vi "test6-AsteriskWildcardStatusRegistration.vi"(8 "error in (no error)":errorcluster, 11 "TestCase in":refnum<class "testcase-CSMBroadcast.lvclass">) -> (0 "error out":errorcluster, 3 "TestCase out":refnum<class "testcase-CSMBroadcast.lvclass">)   [LabVIEW 2017, in "testcase-CSMBroadcast.lvclass"]
uses:
  testcase-CSMBroadcast.lvclass
  0c20cacf-7d77-4f8e-aec5-f22e7d09936d.vi
  26de337d-8090-412f-9da5-e117a55d4726.vi
  de10340a-d592-45ad-b055-7fa7b377c551.vi
  e3eae2f8-d8ce-4adb-8167-9a417250fce1.vi
  a4d00e00-a9ed-4631-bf53-269bf71f16fc.vi
  src/user.lib/_NEVSTOP/Communicable State Machine(CSM)/AdvanceAPI/CSM - Revert Arguments-Safe String.vi
  src/user.lib/_NEVSTOP/Communicable State Machine(CSM)/_Shared/Trim Single-line Text.vi
  src/user.lib/_NEVSTOP/Communicable State Machine(CSM)/AdvanceAPI/CSM - Make String Arguments Safe.vi
  src/user.lib/_NEVSTOP/Communicable State Machine(CSM)/AdvanceAPI/CSM - Break Down Multiple States String.vi
  src/user.lib/_NEVSTOP/Communicable State Machine(CSM)/AdvanceAPI/CSM - Compact Multiple States.vi
  src/user.lib/_NEVSTOP/Communicable State Machine(CSM)/AdvanceAPI/CSM - Keywords.vi
  src/user.lib/_NEVSTOP/Communicable State Machine(CSM)/AdvanceAPI/CSM - Set Module Attribute.vi
  src/user.lib/_NEVSTOP/Communicable State Machine(CSM)/AdvanceAPI/CSM - Get Module Attribute.vi
  <vilib>/addons/_JKI Toolkits/VI Tester/TestCase.llb/TestCase.lvclass
  src/user.lib/_NEVSTOP/Communicable State Machine(CSM)/Communicable State Machine.lvlib
  C:/Program Files (x86)/National Instruments/LabVIEW 2017/vi.lib/addons/_JKI Toolkits/VI Tester/TestCase.llb/TestCase.lvclass
panel:
  out "Execution Times":i32
  out "State History":string
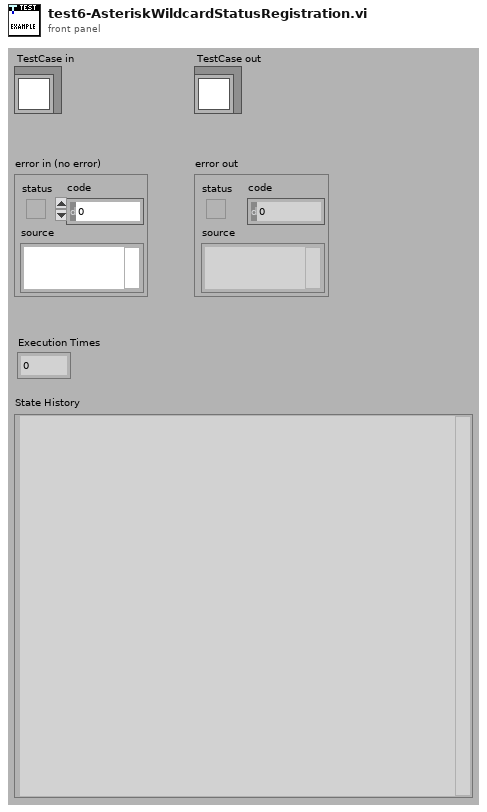
[diagram p1: front panel]
types:
  T1 = enum32{"Invalid", "Standard", "Closed", "Hidden", "Minimized", "Maximized"}
  T2 = enum32{"invalid app kind", "Development System", "Run Time System", "Student Edition", "Embedded LabVIEW", "Evaluation", "Custom"}
  T3 = typedef "Communicable State Machine.lvlib/_CSM_Response Source Message.ctl" = cluster{"‘State":string, "’Arguments":string, "’Error":errorcluster}
  T4 = cluster{"Current VI Reference":refnum<vi>, "Close Panel on Exit?":bool}
  T5 = cluster{"Core":cluster{"Current VI Reference":refnum<vi>, "Close Panel on Exit?":bool}, "Your Boolean data":bool, "Your string data":string, "TestData":i32}
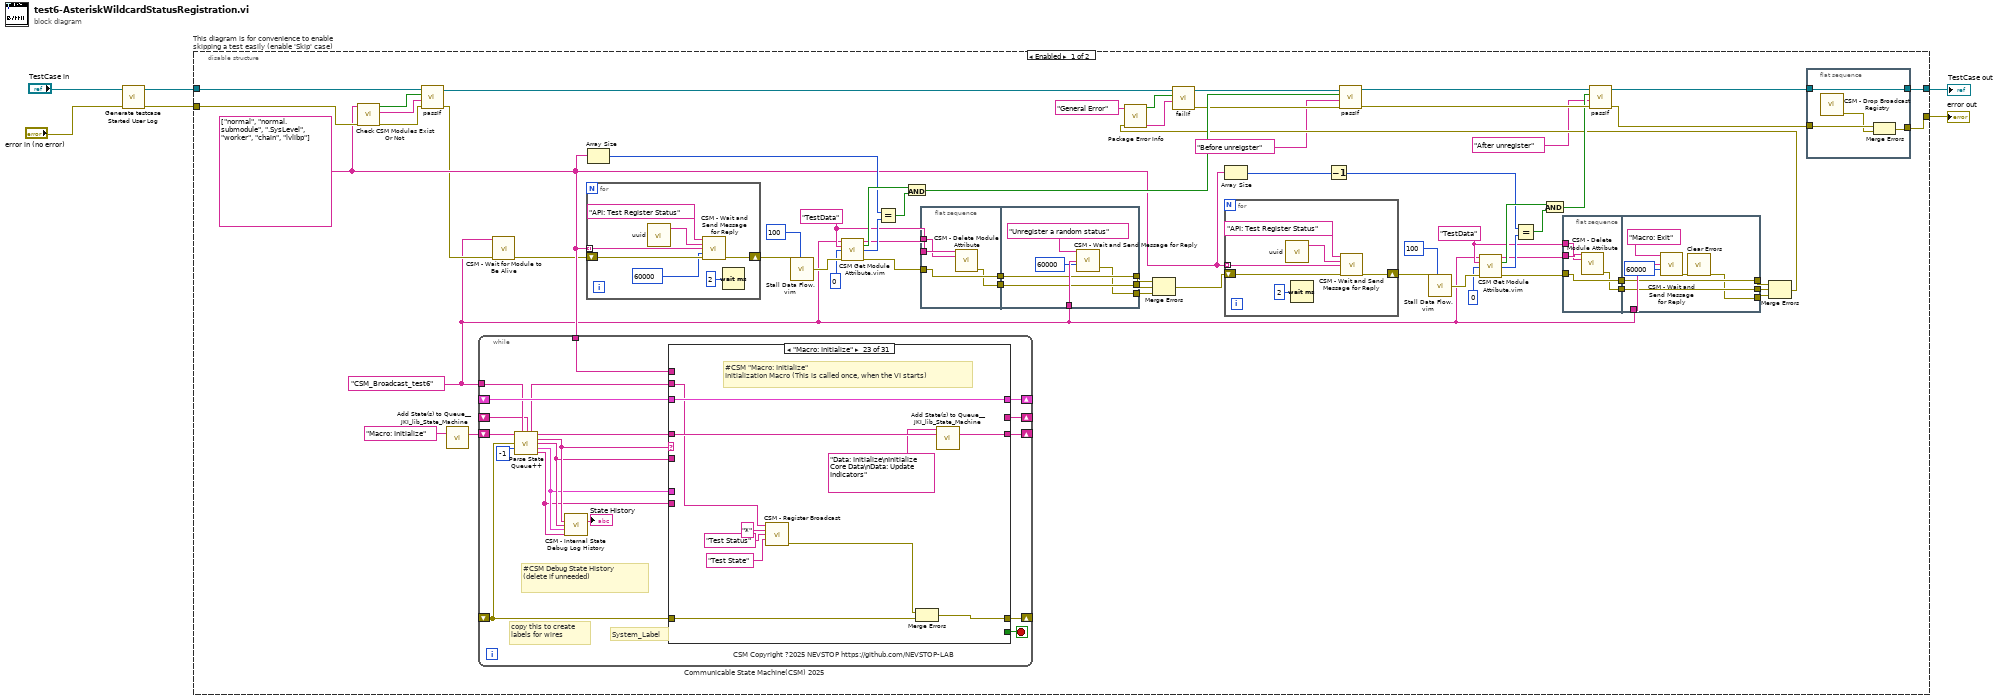
[diagram p0: block diagram]
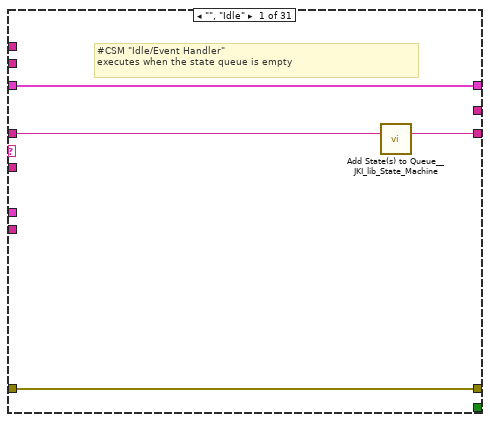
[diagram p2: hidden frame]
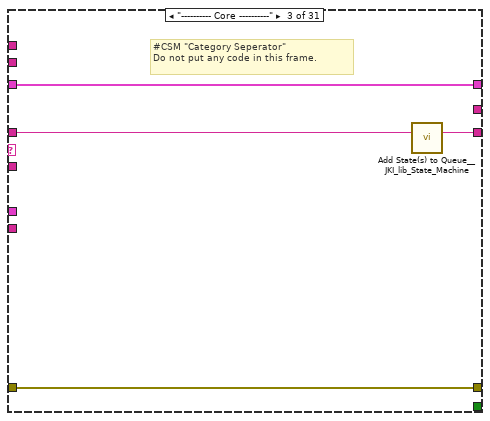
[diagram p4: hidden frame]
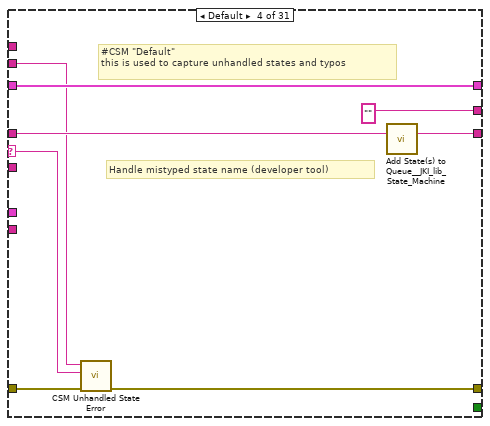
[diagram p5: hidden frame]
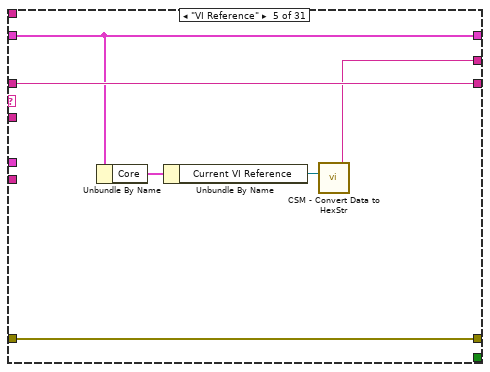
[diagram p6: hidden frame]
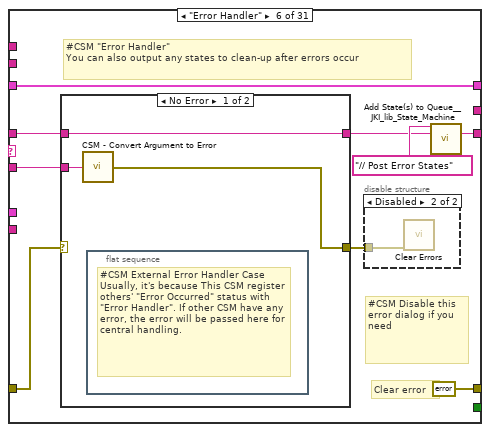
[diagram p7: hidden frame]
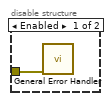
[diagram p8: hidden frame]
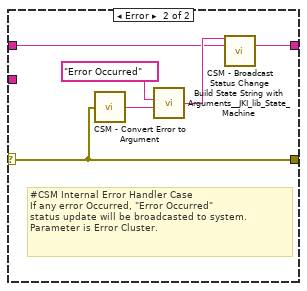
[diagram p9: hidden frame]
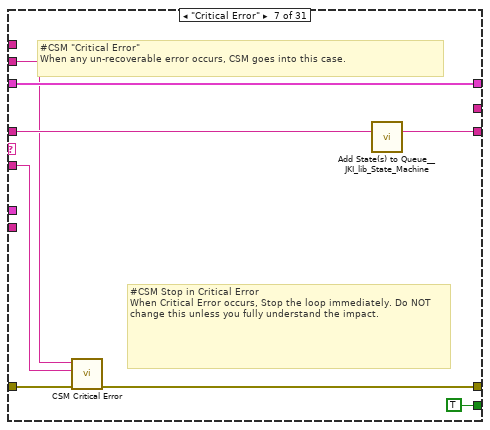
[diagram p10: hidden frame]
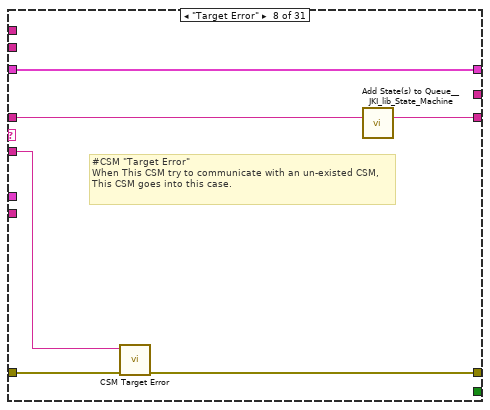
[diagram p11: hidden frame]
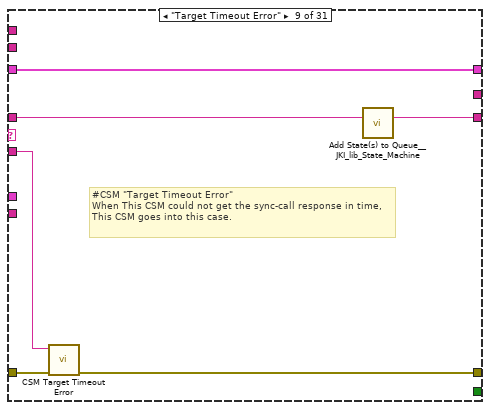
[diagram p12: hidden frame]
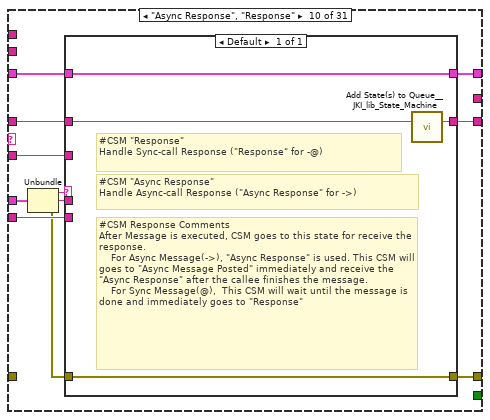
[diagram p13: hidden frame]
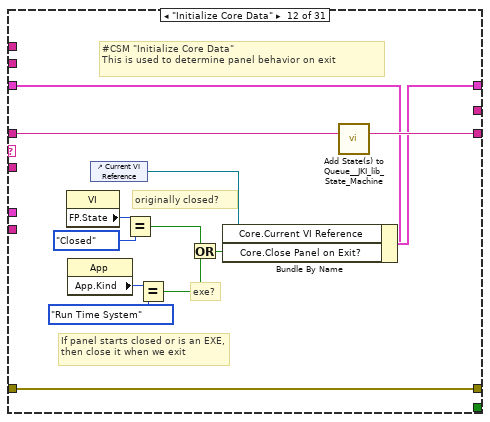
[diagram p15: hidden frame]
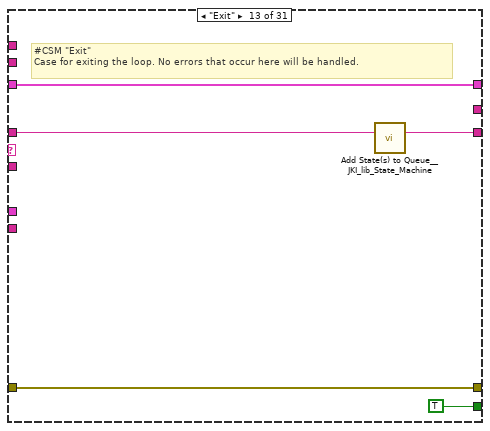
[diagram p16: hidden frame]
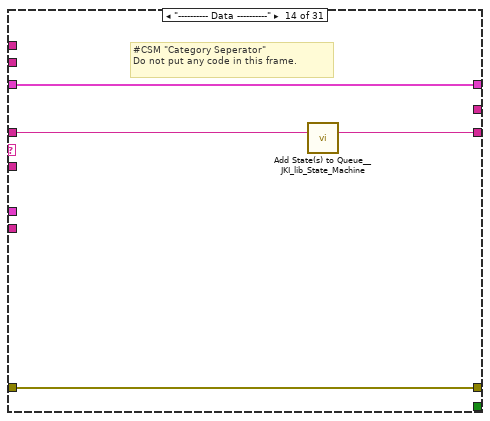
[diagram p17: hidden frame]
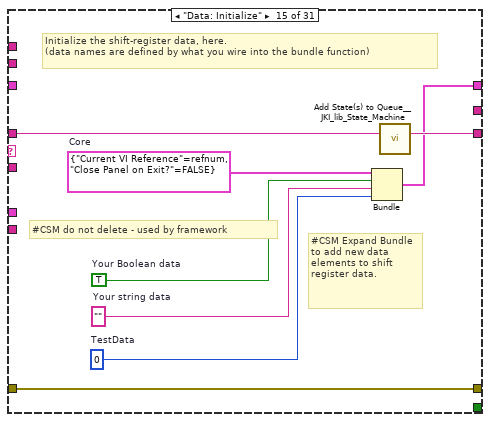
[diagram p18: hidden frame]
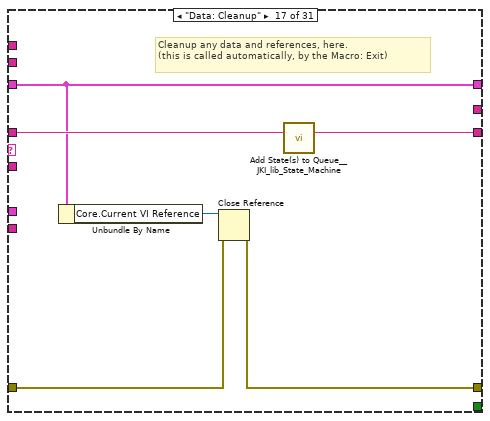
[diagram p20: hidden frame]
diagram:
  n1 = call "Generate testcase Started User Log.vi"("Error In"="error in (no error)") -> ("error out"=w1:errorcluster)  [unwired: 10 in]
  n2 = disable-structure "This diagram is for convenience to enable skipping a test easily (enable 'Skip' case)" shown="Enabled" {
    disable-tunnel: "TestCase in" -> [w24 w425]
    disable-tunnel: [w19 w423] -> w2
    disable-tunnel: [w18 w424] -> w4
    disable-tunnel: w1 -> [w23 w422]
    frame Enabled {
      w33 = "TestData" ("Attribute")
      w55 = "TestData" ("Attribute")
      w6 = "CSM_Broadcast_test6" ("Name (\"\" to Use UUID)")
      w22 = string[] ["normal", "normal.submodule", ".SysLevel", "worker", "chain", "lvlibp"]
      n3 = call "Check CSM Modules Exist Or Not.vi"("error in"=w23, "CSM names in"=w22) -> ("error out"=w25:errorcluster, "Debug string"=w26:string, "All Modules Exist?"=w27:bool)  [unwired: 7 in]
      n4 = call-dynamic "passIf.vi"("error in (no error)"=w25, "message (\"\")"=w26, "pass"=w27, "TestCase in"=w24) -> ("error out"=w8:errorcluster, "TestCase out"=w16:refnum<class "testcase-CSMBroadcast.lvclass">)  [unwired: 6 in]
      n5 = call <vilib>:"Add State(s) to Queue__JKI_lib_State_Machine.vi"("State(s) in (\"\")"="Macro: Initialize" ("Init State(\"Macro: Initialize\")")) -> ("States Out"=w66:string)  [unwired: 14 in]
      n6 = while "Communicable State Machine(CSM) 2025" {
        shift-right: [w112] -> _
        shift-left: _ -> [w111]
        shift-right: [w115] -> _
        shift-left: _ -> [w110]
        shift-right: [w114] -> _
        shift-left: w66 -> [w116]
        tunnel: w6 -> [w108]
        shift-right: [w109] -> _
        shift-left: _ -> [w102]
        tunnel: w22 -> [w99]
        stop <- w113 stop-if-true
        # "#CSM Debug State History\n(delete if unneeded)"
        # "copy this to create labels for wires"
        # "System_Label"
        # "CSM Copyright ?2025 NEVSTOP https://github.com/NEVSTOP-LAB"
        n7 = call "Parse State Queue++.vi"("State Queue"=w116, "Name (\"\" to Use UUID)"=w108, "Response Arguments"=w102, "Previous Error"=w110, "Dequeue (1 ms)"=-1 ("Timeout")) -> ("Name Used"=w103:string, "Remaining States"=w117:string, "Current State"=w107:string, "Arguments"=w106:string, "Additional Information"=w105:T3, "Source CSM"=w104:string)  [unwired: 5 in]
        n8 = call "CSM - Internal State Debug Log History.vi"("State"=w107, "Arguments (\"\")"=w106, ">> Response Source Message >>"=w105, "Source (\"\")"=w104) -> ("Debug Log"=→"State History":string)  [unwired: 11 in]
        n9 = case shown="\"Macro: Initialize\"" w107 {
          selector: w107 -> [_ _ _ w131 _ _ _ _ _ _ _ _ _ _ _ _ _ _ _ _ _ _ _ _ _ _ _ _ _ _ _]
          tunnel: w117 -> [w118 w123 w128 w135 w141 w147 w168 w174 w180 w188 w199 w213 w218 w222 w230 w232 w239 w243 w247 w253 w268 w337 w348 w361 w363 w367 w372 w379 w383 w394 w414]
          tunnel: w106 -> [_ _ _ _ _ w146 w164 w173 w178 w187 _ _ _ _ _ _ _ _ _ w248 w262 _ _ _ _ _ w370 _ _ _ _]
          tunnel: w111 -> [w119 w122 w125 w133 w140 w150 w169 w175 w181 w190 w198 w206 w216 w219 _ w231 w234 w240 w245 w251 w264 w334 w345 w358 w362 w366 w371 w376 w380 w386 w400]
          tunnel: [w120 w124 w126 w129 w142 errorcluster {"status"=FALSE, "code"=0, "source"=""} ("error out") w165 w171 w177 w193 w200 w210 w215 w220 w227 w233 w235 w241 w244 w249 w265 w335 w339 w350 w364 w368 w373 w377 w381 w388 w402] -> w115
          tunnel: w110 -> [w120 w124 w126 w136 w142 w148 w170 w172 w179 _ w200 w210 w215 w220 w227 w233 w236 w241 w244 w250 w266 w335 w346 w359 w364 w368 w373 w377 w381 w392 w412]
          tunnel: [w121 w123 w127 w134 w141 w143 w167 w176 w182 w189 w199 w212 w217 w221 w229 w232 w238 w242 w246 w252 w267 w336 w347 w360 w363 w367 w372 w378 w382 w393 w413] -> w114
          tunnel: [_ _ _ _ _ _ TRUE _ _ _ _ _ TRUE _ _ _ _ _ _ _ _ _ _ _ _ _ _ _ _ _ _] -> w113
          tunnel: [w119 w122 w125 w133 w140 w150 w169 w175 w181 w191 w198 w211 w216 w219 w228 w231 w234 w240 w245 w251 w264 w334 w345 w358 w362 w366 w371 w376 w380 w390 w398] -> w112
          tunnel: w104 -> [_ _ _ _ _ _ _ _ _ w185 _ _ _ _ _ _ _ _ _ _ _ _ _ _ _ _ _ _ _ _ _]
          tunnel: w105 -> [_ _ _ _ _ _ _ _ _ w192 _ _ _ _ _ _ _ _ _ _ _ _ _ _ _ _ _ _ _ _ _]
          tunnel: [_ _ _ "" w137 _ _ _ _ _ _ _ _ _ _ _ _ _ _ _ _ _ _ _ _ "API1 Response" w369 _ _ _ _] -> w109
          tunnel: w103 -> [_ _ _ w130 _ _ w163 _ _ _ _ _ _ _ _ _ _ _ _ _ _ _ w340 w352 _ _ _ _ _ w389 w409]
          tunnel: w99 -> [_ _ _ _ _ _ _ _ _ _ _ _ _ _ _ _ _ _ _ _ _ _ _ _ _ _ _ _ _ _ w405]
          frame "", "Idle" {
            # "#CSM \"Idle/Event Handler\"\nexecutes when the state queue is empty"
            n10 = call <vilib>:"Add State(s) to Queue__JKI_lib_State_Machine.vi"("State(s) in (\"\")"=w118) -> ("States Out"=w121:string)  [unwired: 14 in]
          }
          frame "CSM Documentation" {
            # "#CSM README FIRST\n\nCommunicable State Machine(CSM) is a LabVIEW application framework that builds upon JKI State Machine(JKISM). It follows the pattern of JKISM and extends the keywords to describe message communication between modules, including concepts such as Sync-Message, Async-Message, Subscription/Unsubscription of status - essential elements for creating reusable code modules. For more information, please visit the CSM wiki: https://nevstop-lab.github.io/CSM-Wiki/\n\nFor instructions on JKI State Machine, visit: http://jki.net/state-machine/\nFor information about CSM, visit: https://github.com/NEVSTOP-LAB"
            # "#CSM \"Documentation\"\nCase for holding CSM Documenation"
          }
          frame "---------- Core ----------" {
            # "#CSM \"Category Seperator\"\nDo not put any code in this frame."
            n11 = call <vilib>:"Add State(s) to Queue__JKI_lib_State_Machine.vi"("State(s) in (\"\")"=w128) -> ("States Out"=w127:string)  [unwired: 14 in]
          }
          frame Default {
            # "#CSM \"Default\"\nthis is used to capture unhandled states and typos"
            # "Handle mistyped state name (developer tool)"
            n12 = call "CSM Unhandled State Error.vi"("error in (no error)"=w136, "Undefined State"=w131, "CSM Name"=w130) -> ("error out"=w129:errorcluster)  [unwired: 8 in]
            n13 = call <vilib>:"Add State(s) to Queue__JKI_lib_State_Machine.vi"("State(s) in (\"\")"=w135) -> ("States Out"=w134:string)  [unwired: 14 in]
          }
          frame "VI Reference" {
            n14 = Unbundle By Name(w140) -> ("Core"=w139:T4)
            n15 = Unbundle By Name(w139) -> ("Current VI Reference"=w138:refnum<vi>)
            n16 = call "CSM - Convert Data to HexStr.vi"("Variant"=w138) -> ("HEX String (0-9,A-F)"=w137:string)  [unwired: 8 in]
          }
          frame "Error Handler" {
            # "#CSM Disable this error dialog if you need"
            # "#CSM \"Error Handler\"\nYou can also output any states to clean-up after errors occur"
            # "Clear error"
            n17 = case shown="No Error" w148 {
              selector: w148 -> [_ w157]
              tunnel: [w156 w159] -> w144
              tunnel: w147 -> [w156 w158]
              tunnel: w146 -> [w155 _]
              tunnel: [w154 w157] -> w149
              frame No Error {
                n18 = call "CSM - Convert Argument to Error.vi"("Argument"=w155) -> ("Error"=w154:errorcluster)  [unwired: 4 in]
                n19 = flat-sequence {
                  frame #0 {
                    # "#CSM External Error Handler Case\nUsually, it's because This CSM register others' \"Error Occurred\" status with \"Error Handler\". If other CSM have any error, the error will be passed here for central handling."
                  }
                }
              }
              frame Error {
                # "#CSM Internal Error Handler Case \nIf any error Occurred, \"Error Occurred\" \nstatus update will be broadcasted to system.\nParameter is Error Cluster."
                n20 = call "CSM - Convert Error to Argument.vi"("Error"=w157) -> ("Argument"=w161:string)  [unwired: 4 in]
                n21 = call <vilib>:"Build State String with Arguments__JKI_lib_State_Machine.vi"("Arguments (\"\")"=w161, "State"="Error Occurred" ("Status with Arguments")) -> ("State with Arguments"=w160:string)  [unwired: 4 in]
                n22 = call "CSM - Broadcast Status Change.vi"("Status With Arguments"=w160, "State Queue"=w158) -> ("Remaining States"=w159:string)  [unwired: 13 in]
              }
            }
            n23 = disable-structure shown="Disabled" {
              disable-tunnel: w149 -> [w152 w153]
              frame Enabled {
                n24 = call <vilib>:"General Error Handler.vi"("error in (no error)"=w152) -> ()  [unwired: 10 in, 5 out]
              }
              frame Disabled {
                n25 = call <vilib>:"Clear Errors.vi"("error in (no error)"=w153) -> ()  [unwired: 5 in, 2 out]
              }
            }
            n26 = call <vilib>:"Add State(s) to Queue__JKI_lib_State_Machine.vi"("State(s) in Front (\"\")"="// Post Error States", "State(s) in (\"\")"=w144) -> ("States Out"=w143:string)  [unwired: 13 in]
          }
          frame "Critical Error" {
            # "#CSM Stop in Critical Error\nWhen Critical Error occurs, Stop the loop immediately. Do NOT change this unless you fully understand the impact."
            # "#CSM \"Critical Error\"\nWhen any un-recoverable error occurs, CSM goes into this case."
            n27 = call "CSM Critical Error.vi"("error in (no error)"=w170, "Arugments (As Reason)"=w164, "CSM Name"=w163) -> ("error out"=w165:errorcluster)  [unwired: 8 in]
            n28 = call <vilib>:"Add State(s) to Queue__JKI_lib_State_Machine.vi"("State(s) in (\"\")"=w168) -> ("States Out"=w167:string)  [unwired: 14 in]
          }
          frame "Target Error" {
            # "#CSM \"Target Error\"\nWhen This CSM try to communicate with an un-existed CSM, This CSM goes into this case."
            n29 = call "CSM Target Error.vi"("error in (no error)"=w172, "Arguments (As CSM Name)"=w173) -> ("error out"=w171:errorcluster)  [unwired: 9 in]
            n30 = call <vilib>:"Add State(s) to Queue__JKI_lib_State_Machine.vi"("State(s) in (\"\")"=w174) -> ("States Out"=w176:string)  [unwired: 14 in]
          }
          frame "Target Timeout Error" {
            # "#CSM \"Target Timeout Error\"\nWhen This CSM could not get the sync-call response in time, This CSM goes into this case."
            n31 = call "CSM Target Timeout Error.vi"("error in (no error)"=w179, "Arguments (As CSM Name)"=w178) -> ("error out"=w177:errorcluster)  [unwired: 9 in]
            n32 = call <vilib>:"Add State(s) to Queue__JKI_lib_State_Machine.vi"("State(s) in (\"\")"=w180) -> ("States Out"=w182:string)  [unwired: 14 in]
          }
          frame "Async Response", "Response" {
            n33 = Unbundle(w192) -> ("‘State"=w186:string, "’Arguments"=w184:string, "’Error"=w183:errorcluster)
            n34 = case shown="Default" w186 {
              tunnel: [w197] -> w193
              tunnel: w183 -> [w197]
              tunnel: [w196] -> w191
              tunnel: w190 -> [w196]
              tunnel: [w194] -> w189
              tunnel: w188 -> [w195]
              tunnel: w187 -> [_]
              tunnel: w185 -> [_]
              tunnel: w184 -> [_]
              frame Default {
                # "#CSM Response Comments\nAfter Message is executed, CSM goes to this state for receive the response.\n    For Async Message(->), \"Async Response\" is used. This CSM will goes to \"Async Message Posted\" immediately and receive the \"Async Response\" after the callee finishes the message.\n    For Sync Message(@),  This CSM will wait until the message is done and immediately goes to \"Response\""
                # "#CSM \"Async Response\"\nHandle Async-call Response (\"Async Response\" for ->)"
                # "#CSM \"Response\"\nHandle Sync-call Response (\"Response\" for -@)"
                n35 = call <vilib>:"Add State(s) to Queue__JKI_lib_State_Machine.vi"("State(s) in (\"\")"=w195) -> ("States Out"=w194:string)  [unwired: 14 in]
              }
            }
          }
          frame "Async Message Posted" {
            # "#CSM \"Async Message Posted\"\nAfter Async Message is posted (-> or ->| ), CSM goes to this state for post-action.\nYou can use Argument - State to tell which Async Message is called."
          }
          frame "Initialize Core Data" {
            # "#CSM \"Initialize Core Data\"\nThis is used to determine panel behavior on exit"
            # "originally closed?"
            # "exe?"
            # "If panel starts closed or is an EXE, then close it when we exit"
            n36 = property class="VI"() -> ("FP.State"=w203:T1)  [unwired: 2 in, 2 out]
            n37 = property class="App"() -> ("App.Kind"=w209:T2)  [unwired: 2 in, 2 out]
            n38 = control-ref of="Current VI Reference"() -> (w204:refnum<vi>)
            n39 = Equal?(x=w203, y=T1."Closed" ("Front Panel Window:State")) -> (x = y?=w201:bool)
            n40 = Equal?(x=w209, y=T2."Run Time System" ("Application:Kind")) -> (x = y?=w207:bool)
            n41 = Or(x=w201, y=w207) -> (x .or. y?=w205:bool)
            n42 = Bundle By Name(cluster=w206, "Core.Current VI Reference"=w204, "Core.Close Panel on Exit?"=w205) -> (w211:T5)
            n43 = call <vilib>:"Add State(s) to Queue__JKI_lib_State_Machine.vi"("State(s) in (\"\")"=w213) -> ("States Out"=w212:string)  [unwired: 14 in]
          }
          frame "Exit" {
            # "#CSM \"Exit\"\nCase for exiting the loop. No errors that occur here will be handled."
            n44 = call <vilib>:"Add State(s) to Queue__JKI_lib_State_Machine.vi"("State(s) in (\"\")"=w218) -> ("States Out"=w217:string)  [unwired: 14 in]
          }
          frame "---------- Data ----------" {
            # "#CSM \"Category Seperator\"\nDo not put any code in this frame."
            n45 = call <vilib>:"Add State(s) to Queue__JKI_lib_State_Machine.vi"("State(s) in (\"\")"=w222) -> ("States Out"=w221:string)  [unwired: 14 in]
          }
          frame "Data: Initialize" {
            w223 = 0  # TestData
            w224 = T4 {"Current VI Reference"=refnum, "Close Panel on Exit?"=FALSE}  # Core
            w226 = TRUE  # Your Boolean data
            w225 = ""  # Your string data
            # "#CSM do not delete - used by framework"
            # "#CSM Expand Bundle to add new data elements to shift register data."
            # "Initialize the shift-register data, here.\n(data names are defined by what you wire into the bundle function)"
            n46 = Bundle("Core"=w224, "Your Boolean data"=w226, "Your string data"=w225, "TestData"=w223) -> (w228:T5)  [unwired: 1 in]
            n47 = call <vilib>:"Add State(s) to Queue__JKI_lib_State_Machine.vi"("State(s) in (\"\")"=w230) -> ("States Out"=w229:string)  [unwired: 14 in]
          }
          frame "Data: Update Indicators" {
          }
          frame "Data: Cleanup" {
            # "Cleanup any data and references, here.\n(this is called automatically, by the Macro: Exit)"
            n48 = Unbundle By Name(w234) -> ("Core.Current VI Reference"=w237:refnum<vi>)
            n49 = Close Reference(reference=w237, error in (no error)=w236) -> (error out=w235:errorcluster)
            n50 = call <vilib>:"Add State(s) to Queue__JKI_lib_State_Machine.vi"("State(s) in (\"\")"=w239) -> ("States Out"=w238:string)  [unwired: 14 in]
          }
          frame "---------- UI ----------" {
            # "#CSM \"Category Seperator\"\nDo not put any code in this frame."
            n51 = call <vilib>:"Add State(s) to Queue__JKI_lib_State_Machine.vi"("State(s) in (\"\")"=w243) -> ("States Out"=w242:string)  [unwired: 14 in]
          }
          frame "UI: Initialize" {
            # "#CSM \"UI: Initialize\"\nInitialize the User Interface, here.\n(this is called automatically, by the Macro: Init)"
            n52 = call <vilib>:"Add State(s) to Queue__JKI_lib_State_Machine.vi"("State(s) in (\"\")"=w247) -> ("States Out"=w246:string)  [unwired: 14 in]
          }
          frame "UI: Cursor Set" {
            # "#CSM \"UI: Cursor Set\"\nSet and Unset Cursor Busy.\n(Usage: \"UI: Cursor Set >> Busy|Idle\")"
            # "Argument"
            n53 = disable-structure shown="TARGET_TYPE!=Windows" {
              disable-tunnel: w250 -> [w256 w261]
              disable-tunnel: [w255 w261] -> w249
              disable-tunnel: w248 -> [w254 _]
              frame condition #0 (active) {
                n54 = case shown="\"Idle\", Default" w254 {
                  tunnel: w256 -> [w258 w260]
                  tunnel: [w257 w259] -> w255
                  frame "Idle", Default {
                    n55 = call <vilib>:"Unset Busy.vi"("error in (no error)"=w258) -> ("error out"=w257:errorcluster)  [unwired: 10 in]
                  }
                  frame "Busy" {
                    n56 = call <vilib>:"Set Busy.vi"("error in (no error)"=w260) -> ("error out"=w259:errorcluster)  [unwired: 9 in, 1 out]
                  }
                }
              }
              frame condition #1 {
              }
            }
            n57 = call <vilib>:"Add State(s) to Queue__JKI_lib_State_Machine.vi"("State(s) in (\"\")"=w253) -> ("States Out"=w252:string)  [unwired: 14 in]
          }
          frame "UI: Front Panel State" {
            # "#CSM \"UI: Front Panel State\"\nSet Front Panel Open or Closed\n(Usage: \"UI: Front Panel State >> Open|Close\")"
            # "Argument"
            n58 = Unbundle By Name(w264) -> ("Core.Current VI Reference"=w263:refnum<vi>)
            n59 = call <vilib>:"Add State(s) to Queue__JKI_lib_State_Machine.vi"("State(s) in (\"\")"=w268) -> ("States Out"=w267:string)  [unwired: 14 in]
            n60 = case shown="\"Close\", \"Closed\"" w262 {
              tunnel: w266 -> [w274 w289 w300 w313 w326]
              tunnel: [w276 w290 w302 w315 w328] -> w265
              tunnel: w263 -> [w275 w287 w301 w314 w327]
              frame "Open", "Standard", Default {
                w269 = T1."Standard" ("State")
                n61 = property class="VI"(reference=w275, error in=w274) -> (reference out=w272:refnum<vi>, error out=w273:errorcluster, "FP.State"=w271:T1)
                n62 = Not Equal?(x=w271, y=w269) -> (x != y?=w270:bool)
                n63 = case shown="True" w270 {
                  tunnel: [w280 w282] -> w276
                  tunnel: w273 -> [w279 w282]
                  tunnel: w272 -> [w278 _]
                  tunnel: w269 -> [w277 _]
                  frame True {
                    n64 = invoke class="VI" method="FP.Open"(reference=w278, error in=w279, "Activate"=TRUE, "State"=w277) -> (error out=w280:errorcluster)  [unwired: 1 in, 4 out]
                  }
                  frame False {
                  }
                }
              }
              frame "Close", "Closed" {
                n65 = property class="VI"(reference=w287, error in=w289) -> (reference out=w286:refnum<vi>, error out=w288:errorcluster, "FP.State"=w284:T1)
                n66 = Not Equal?(x=w284, y=T1."Closed" ("Front Panel Window:State")) -> (x != y?=w283:bool)
                n67 = case shown="False" w283 {
                  tunnel: [w291 w294] -> w290
                  tunnel: w288 -> [w291 w293]
                  tunnel: w286 -> [_ w292]
                  frame False {
                  }
                  frame True {
                    n68 = invoke class="VI" method="FP.Close"(reference=w292, error in=w293) -> (error out=w294:errorcluster)  [unwired: 1 in, 2 out]
                  }
                }
              }
              frame "Hidden", "Hide" {
                w295 = T1."Hidden" ("State")
                n69 = property class="VI"(reference=w301, error in=w300) -> (reference out=w298:refnum<vi>, error out=w299:errorcluster, "FP.State"=w297:T1)
                n70 = Not Equal?(x=w297, y=w295) -> (x != y?=w296:bool)
                n71 = case shown="True" w296 {
                  tunnel: [w306 w307] -> w302
                  tunnel: w299 -> [w305 w307]
                  tunnel: w298 -> [w304 _]
                  tunnel: w295 -> [w303 _]
                  frame True {
                    n72 = invoke class="VI" method="FP.Open"(reference=w304, error in=w305, "State"=w303) -> (error out=w306:errorcluster)  [unwired: 2 in, 4 out]
                  }
                  frame False {
                  }
                }
              }
              frame "Minimize", "Minimized" {
                w308 = T1."Minimized" ("State")
                n73 = property class="VI"(reference=w314, error in=w313) -> (reference out=w311:refnum<vi>, error out=w312:errorcluster, "FP.State"=w310:T1)
                n74 = Not Equal?(x=w310, y=w308) -> (x != y?=w309:bool)
                n75 = case shown="True" w309 {
                  tunnel: [w319 w320] -> w315
                  tunnel: w312 -> [w318 w320]
                  tunnel: w311 -> [w317 _]
                  tunnel: w308 -> [w316 _]
                  frame True {
                    n76 = invoke class="VI" method="FP.Open"(reference=w317, error in=w318, "State"=w316) -> (error out=w319:errorcluster)  [unwired: 2 in, 4 out]
                  }
                  frame False {
                  }
                }
              }
              frame "Maximize", "Maximized" {
                w321 = T1."Maximized" ("State")
                n77 = property class="VI"(reference=w327, error in=w326) -> (reference out=w324:refnum<vi>, error out=w325:errorcluster, "FP.State"=w323:T1)
                n78 = Not Equal?(x=w323, y=w321) -> (x != y?=w322:bool)
                n79 = case shown="True" w322 {
                  tunnel: [w332 w333] -> w328
                  tunnel: w325 -> [w331 w333]
                  tunnel: w324 -> [w330 _]
                  tunnel: w321 -> [w329 _]
                  frame True {
                    n80 = invoke class="VI" method="FP.Open"(reference=w330, error in=w331, "State"=w329) -> (error out=w332:errorcluster)  [unwired: 2 in, 4 out]
                  }
                  frame False {
                  }
                }
              }
            }
          }
          frame "---------- Macro ----------" {
            # "#CSM \"Category Seperator\"\nDo not put any code in this frame."
            n81 = call <vilib>:"Add State(s) to Queue__JKI_lib_State_Machine.vi"("State(s) in (\"\")"=w337) -> ("States Out"=w336:string)  [unwired: 14 in]
          }
          frame "Macro: Initialize" {
            # "#CSM \"Macro: Initialize\"\nInitialization Macro (This is called once, when the VI starts)"
            n82 = call "CSM - Register Broadcast.vi"("CSM Name(Empty for Broadcast Event)"=w340, "Source CSM Name (* as Default)"="*", "Trigger"="Test Status" ("Status"), "API (If \"\", Same as Trigger)"="Test State" ("Response Message (If \"\", Same as Source Message)")) -> ("error out"=w338:errorcluster)  [unwired: 10 in, 1 out]
            n83 = Merge Errors(w338, w346) -> (w339:errorcluster)
            n84 = call <vilib>:"Add State(s) to Queue__JKI_lib_State_Machine.vi"("State(s) in Front (\"\")"="Data: Initialize\nInitialize Core Data\nData: Update Indicators", "State(s) in (\"\")"=w348) -> ("States Out"=w347:string)  [unwired: 13 in]
          }
          frame "Macro: Exit" {
            # "#CSM \"Macro: Exit\"\nExit Macro (This is called once, when the VI exits)"
            n85 = call "CSM - Unregister Broadcast.vi"("CSM Name(Empty for Broadcast Event)"=w352, "Source CSM Name (* as Default)"="*", "Trigger"="Test Status" ("Status"), "API (\"*\" as Default)"="Test State" ("Response Message (If \"\", Same as Source Message)")) -> ("error out"=w349:errorcluster)  [unwired: 10 in, 1 out]
            n86 = call <vilib>:"Add State(s) to Queue__JKI_lib_State_Machine.vi"("State(s) in Front (\"\")"="//Exit Sub-Modules ", "State(s) at Back (\"\")"="Data: Cleanup\nExit") -> ("States Out"=w356:string)  [unwired: 13 in]
            n87 = Merge Errors(w349, w359) -> (w350:errorcluster)
            n88 = call <vilib>:"Add State(s) to Queue__JKI_lib_State_Machine.vi"("State(s) in Front (\"\")"=w356, "State(s) in (\"\")"=w361) -> ("States Out"=w360:string)  [unwired: 13 in]
          }
          frame "---------- API ----------" {
            # "#CSM \"Category Seperator\"\nDo not put any code in this frame."
          }
          frame "API: API1" {
            # "#CSM API Example\nCopy/Rename this case for your own API"
            # "#CSM Response\nConnect this to return the response of your API"
            # "#CSM >> Msg/Rep's CSM >>\nIf you need to tell who triggered this state , use this string. If it's this case itself, this string is \"\"."
            # "#CSM >> Arguments >>\nDeal with the parameter if any"
          }
          frame "API: API2" {
            # "#CSM API Example\nCopy/Rename this case for your own API"
            # "unpack Hex String  to Variant\nif complex parameter is needed."
            n89 = call "CSM - Convert HexStr to Data.vi"("HEX String"=w370) -> ()  [unwired: 7 in, 2 out]
            n90 = disable-structure shown="Disabled" {
              disable-tunnel: [w374 "API2 Response"] -> w369
              frame Disabled {
                # "pack variant to hexstr \nif complex response is needed."
                # "complex Response"
                n91 = call "CSM - Convert Data to HexStr.vi"() -> ("HEX String (0-9,A-F)"=w374:string)  [unwired: 9 in]
              }
              frame Enabled {
              }
            }
          }
          frame "---------- Action ----------" {
            # "#CSM \"Category Seperator\"\nDo not put any code in this frame."
            n92 = call <vilib>:"Add State(s) to Queue__JKI_lib_State_Machine.vi"("State(s) in (\"\")"=w379) -> ("States Out"=w378:string)  [unwired: 14 in]
          }
          frame "Action: action1" {
            # "#CSM \"Internal State\"\nThis category is used for holding internal states"
            n93 = call <vilib>:"Add State(s) to Queue__JKI_lib_State_Machine.vi"("State(s) in (\"\")"=w383) -> ("States Out"=w382:string)  [unwired: 14 in]
          }
          frame "Test State" {
            n94 = Unbundle By Name(w386) -> ("TestData"=w391:i32)
            n95 = disable-structure shown="Enabled" {
              frame Disabled {
                n96 = feedback #1(0 ("y")) -> (w396:i32)
                n97 = Increment(x=w396) -> (x+1=w395:i32)
                "Execution Times" <- w395
                n98 = feedback-in #1(w395) -> ()
              }
              frame Enabled {
              }
            }
            n99 = Increment(x=w391) -> (x+1=w384:i32)
            n100 = Bundle By Name(cluster=w386, "TestData"=w384) -> (w390:T5)
            n101 = call "CSM Set Module Attribute.vim"("CSM Name"=w389, "Attribute"="TestData", "Value"=w384) -> ("error out"=w387:errorcluster)  [unwired: 9 in, 3 out]
            n102 = call <vilib>:"Add State(s) to Queue__JKI_lib_State_Machine.vi"("State(s) in (\"\")"=w394) -> ("States Out"=w393:string)  [unwired: 14 in]
            n103 = Merge Errors(w392, w387) -> (w388:errorcluster)
          }
          frame "Unregister a random status" {
            n104 = Random Number (0-1)() -> (number: 0 to 1=w407:dbl)
            n105 = Array Size(array=w405) -> (size(s)=w408:i32)
            n106 = Multiply(x=w408, y=w407) -> (x*y=w406:dbl)
            n107 = Bundle By Name(cluster=w400, "TestData"=0) -> (w398:T5)
            n108 = Round Toward -Infinity(1:w406) -> (0:w404:dbl)
            n109 = Index Array(array=w405, index=w404) -> (element=w403:string)
            n110 = call "CSM - Unregister Broadcast.vi"("CSM Name(Empty for Broadcast Event)"=w409, "Source CSM Name (* as Default)"=w403, "Trigger"="Test Status" ("Status"), "API (\"*\" as Default)"="Test State" ("Response Message (If \"\", Same as Source Message)")) -> ("error out"=w401:errorcluster)  [unwired: 10 in, 1 out]
            n111 = Merge Errors(w412, w401) -> (w402:errorcluster)
            n112 = call <vilib>:"Add State(s) to Queue__JKI_lib_State_Machine.vi"("State(s) in (\"\")"=w414) -> ("States Out"=w413:string)  [unwired: 14 in]
          }
        }
      }
      n113 = call "CSM - Wait for Module to Be Alive.vi"("CSM Name"=w6, "error in (no error)"=w8) -> ("error out"=w7:errorcluster)  [unwired: 11 in, 2 out]
      n114 = for {
        tunnel: w22 -> [w419] mode=indexing
        shift-right: [w418] -> w64
        shift-left: w7 -> [w417]
        n115 = call "uuid.vi"() -> ("UUID"=w420:string)  [unwired: 11 in]
        n116 = call "CSM - Wait and Send Message for Reply.vi"("State"="API: Test Register Status", "Arguments (\"\")"=w420, "Target Module"=w419, "Wait (5000ms)"=60000, "Error In (No Error)"=w417) -> ("error out"=w418:errorcluster)  [unwired: 7 in, 3 out]
        n117 = Wait (ms)(milliseconds to wait=u32 2) -> ()  [unwired: 1 out]
      }
      n118 = Array Size(array=w22) -> (size(s)=w59:i32)
      n119 = call "Stall Data Flow.vim"("value in"=w64, "milliseconds to wait"=u32 100) -> ("value out"=w63:errorcluster)  [unwired: 1 out]
      n120 = call "CSM Get Module Attribute.vim"("CSM Name"=w6, "Attribute"=w55, "Default Value (Empty Variant)"=0 ("x+1"), "Error In"=w63) -> ("CSM Name (Dup)"=w56:string, "Found"=w61:bool, "Value"=w60:i32, "error out"=w54:errorcluster)  [unwired: 7 in, 1 out]
      n121 = Equal?(x=w59, y=w60) -> (x = y?=w58:bool)
      n122 = And(x=w61, y=w58) -> (x .and. y?=w57:bool)
      n123 = flat-sequence {
        tunnel: w56 -> [w92]
        tunnel: w55 -> [w91]
        tunnel: w54 -> [w90]
        tunnel: [w90] -> w53
        tunnel: [w89] -> w52
        tunnel: w6 -> [w97]
        tunnel: w53 -> [w96]
        tunnel: w52 -> [w95]
        tunnel: [w96] -> w51
        tunnel: [w95] -> w50
        tunnel: [w94] -> w49
        frame #0 {
          n124 = call "CSM - Delete Module Attribute.vi"("CSM Name"=w92, "Attribute"=w91) -> ("error out"=w89:errorcluster)  [unwired: 10 in, 3 out]
        }
        frame #1 {
          n125 = call "CSM - Wait and Send Message for Reply.vi"("State"="Unregister a random status", "Target Module"=w97, "Wait (5000ms)"=60000) -> ("error out"=w94:errorcluster)  [unwired: 9 in, 3 out]
        }
      }
      n126 = Merge Errors(w51, w50, w49) -> (w41:errorcluster)
      n127 = for {
        tunnel: w22 -> [w86] mode=indexing
        shift-right: [w85] -> w47
        shift-left: w41 -> [w84]
        n128 = call "uuid.vi"() -> ("UUID"=w87:string)  [unwired: 11 in]
        n129 = Wait (ms)(milliseconds to wait=u32 2) -> ()  [unwired: 1 out]
        n130 = call "CSM - Wait and Send Message for Reply.vi"("State"="API: Test Register Status", "Arguments (\"\")"=w87, "Target Module"=w86, "Error In (No Error)"=w84) -> ("error out"=w85:errorcluster)  [unwired: 8 in, 3 out]
      }
      n131 = Array Size(array=w22) -> (size(s)=w40:i32)
      n132 = Decrement(x=w40) -> (x-1=w39:i32)
      n133 = call "Stall Data Flow.vim"("value in"=w47, "milliseconds to wait"=u32 100) -> ("value out"=w46:errorcluster)  [unwired: 1 out]
      n134 = call "CSM Get Module Attribute.vim"("CSM Name"=w6, "Attribute"=w33, "Default Value (Empty Variant)"=0 ("x+1"), "Error In"=w46) -> ("CSM Name (Dup)"=w34:string, "Found"=w44:bool, "Value"=w43:i32, "error out"=w32:errorcluster)  [unwired: 7 in, 1 out]
      n135 = Equal?(x=w39, y=w43) -> (x = y?=w42:bool)
      n136 = And(x=w44, y=w42) -> (x .and. y?=w28:bool)
      n137 = flat-sequence {
        tunnel: w34 -> [w75]
        tunnel: w33 -> [w74]
        tunnel: w32 -> [w73]
        tunnel: [w73] -> w36
        tunnel: [w72] -> w35
        tunnel: w6 -> [w81]
        tunnel: w36 -> [w80]
        tunnel: w35 -> [w79]
        tunnel: [w80] -> w31
        tunnel: [w79] -> w30
        tunnel: [w77] -> w29
        frame #0 {
          n138 = call "CSM - Delete Module Attribute.vi"("CSM Name"=w75, "Attribute"=w74) -> ("error out"=w72:errorcluster)  [unwired: 10 in, 3 out]
        }
        frame #1 {
          n139 = call "CSM - Wait and Send Message for Reply.vi"("State"="Macro: Exit", "Target Module"=w81, "Wait (5000ms)"=60000) -> ("error out"=w78:errorcluster)  [unwired: 9 in, 3 out]
          n140 = call <vilib>:"Clear Errors.vi"("error in (no error)"=w78) -> ("error out"=w77:errorcluster)  [unwired: 5 in, 1 out]
        }
      }
      n141 = Merge Errors(w31, w30, w29) -> (w12:errorcluster)
      n142 = call "Package Error Info.vi"("error in"=w12, "String in"="General Error") -> ("packed error info out"=w13:string, "error status"=w17:bool)  [unwired: 8 in]
      n143 = call-dynamic "failIf.vi"("message (\"\")"=w13, "fail"=w17, "TestCase in"=w16) -> ("error out"=w14:errorcluster, "TestCase out"=w15:refnum<class "testcase-CSMBroadcast.lvclass">)  [unwired: 7 in]
      n144 = call-dynamic "passIf.vi"("error in (no error)"=w14, "message (\"\")"="Before unreigster" ("message (\"\")"), "pass"=w57, "TestCase in"=w15) -> ("error out"=w38:errorcluster, "TestCase out"=w37:refnum<class "testcase-CSMBroadcast.lvclass">)  [unwired: 6 in]
      n145 = call-dynamic "passIf.vi"("error in (no error)"=w38, "message (\"\")"="After unregister" ("message (\"\")"), "pass"=w28, "TestCase in"=w37) -> ("error out"=w20:errorcluster, "TestCase out"=w21:refnum<class "testcase-CSMBroadcast.lvclass">)  [unwired: 6 in]
      n146 = flat-sequence {
        tunnel: w20 -> [w71]
        tunnel: [w70] -> w18
        tunnel: w21 -> [w68]
        tunnel: [w68] -> w19
        frame #0 {
          n147 = call "CSM - Drop Broadcast Registry.vi"() -> ("error out"=w69:errorcluster)  [unwired: 15 in]
          n148 = Merge Errors(w71, w69) -> (w70:errorcluster)
        }
      }
    }
    frame Disabled {
      # "skip test result while test is under development"
      n149 = call <vilib>:"skip.vi"("error in (no error)"=w422, "TestCase in"=w425) -> ("error out"=w424:errorcluster, "TestCase out"=w423:refnum<class "testcase-CSMBroadcast.lvclass">)  [unwired: 8 in]
    }
  }
  "error out" <- w4
  "TestCase out" <- w2
